vi "Diode FFT test.vi"() -> ()   [LabVIEW 2016]
uses:
  <vilib>/DAQmx/read.llb/DAQmx Read (Analog DBL 1Chan 1Samp).vi
  <vilib>/DAQmx/create/channels.llb/DAQmx Create Channel (AI-Voltage-Basic).vi
  <vilib>/DAQmx/configure/timing.llb/DAQmx Timing (Sample Clock).vi
  <vilib>/DAQmx/miscellaneous.llb/DAQmx Fill In Error Info.vi
  <vilib>/measure/maspectr.llb/FFT Power Spectrum and PSD for 1 Chan.vi
  <vilib>/measure/NI_MAPro.lvlib
panel:
  out "Waveform Graph":cluster{"f0":dbl, "df":dbl, "magnitude":dbl[]}(graph)
  out "Waveform Chart":waveform(dbl)(graph)
  in  "Stop Button":bool
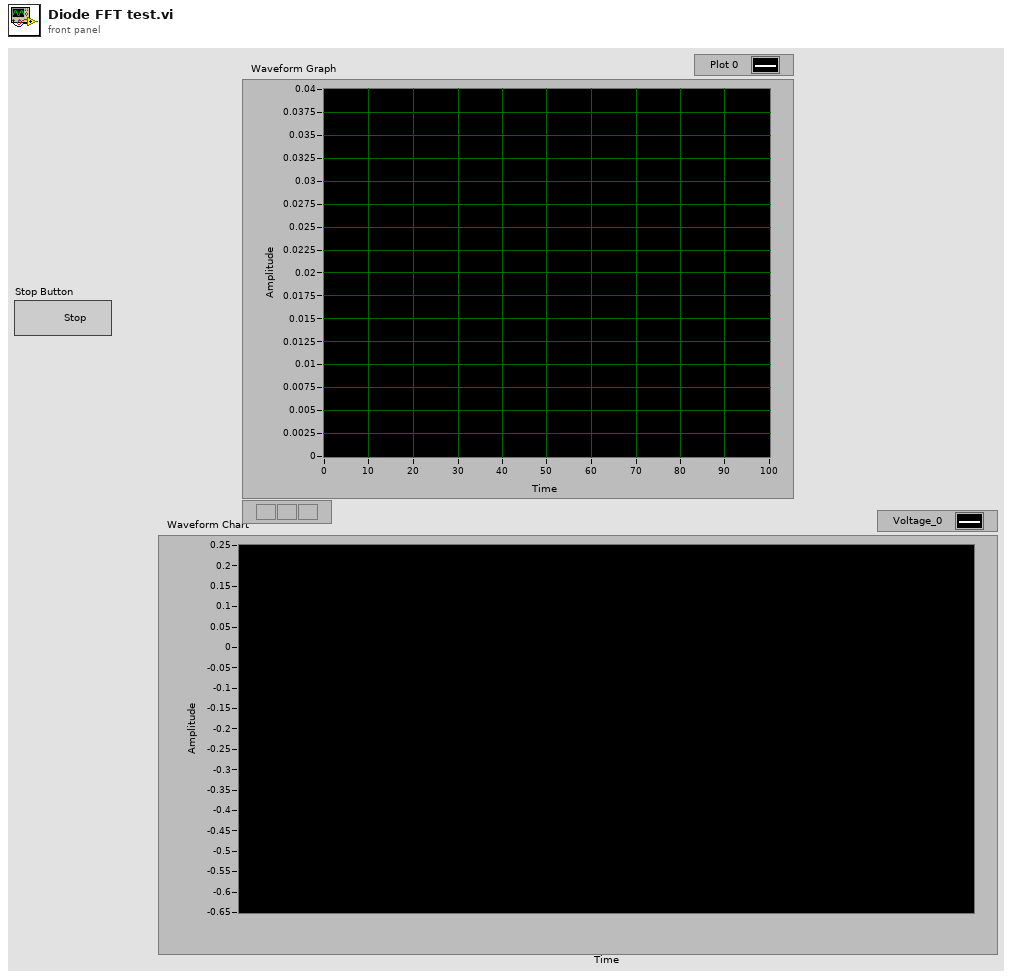
[diagram p1: front panel]
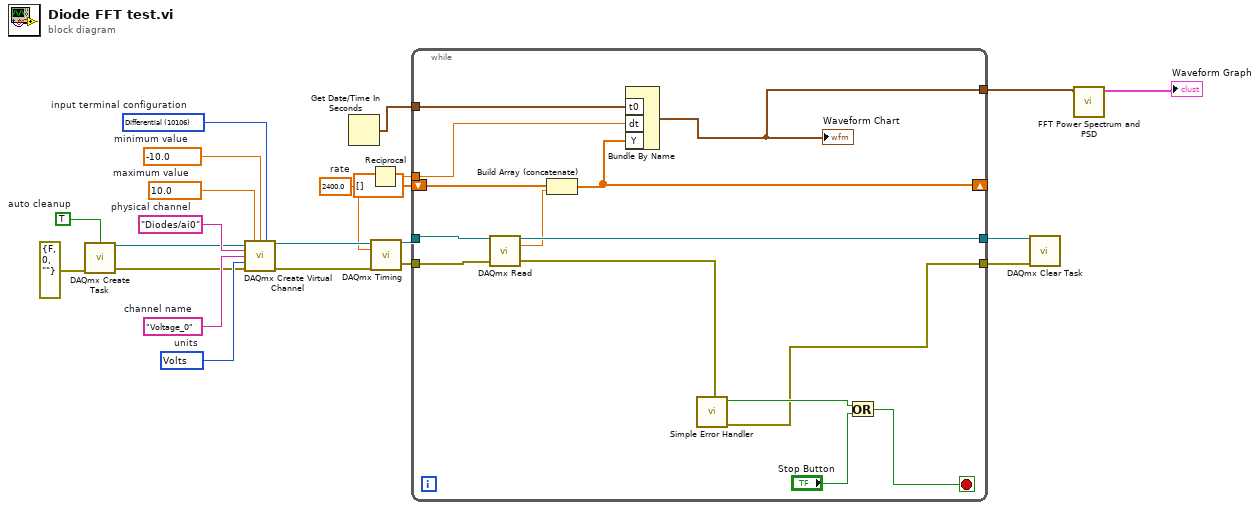
[diagram p0: block diagram]
diagram:
  w5 = 2400.0  # rate
  w13 = 10106 items=["default"=-1, "RSE"=10083, "NRSE"=10078, "Differential"=10106, "Pseudodifferential"=12529]  # input terminal configuration
  w18 = 10348 items=["Volts"=10348, "From Custom Scale"=10065]  # units
  w17 = "Voltage_0"  # channel name
  w14 = -10.0  # minimum value
  w16 = 10.0  # maximum value
  w15 = "Diodes/ai0"  # physical channel
  w20 = TRUE  # auto cleanup
  n1 = call <vilib>:"DAQmx Create Task.vi"("auto cleanup"=w20, "error in"=errorcluster {"status"=FALSE, "code"=0, "source"=""}) -> ("task out"=w11:refnum<k21>, "error out"=w12:errorcluster)  [unwired: 12 in]
  n2 = call-poly <vilib>:"DAQmx Create Virtual Channel.vi"("task in"=w11, "maximum value"=w16, "minimum value"=w14, "input terminal configuration"=w13, "physical channels"=w15, "name to assign"=w17, "units"=w18, "error in"=w12) -> ("task out"=w10:refnum<k21>, "error out"=w8:errorcluster)  [unwired: 6 in]
  n3 = Get Date/Time In Seconds() -> (seconds since 1Jan1904=w6:timestamp)
  n4 = Reciprocal(x=w5) -> (1/x=w4:dbl)
  n5 = call-poly <vilib>:"DAQmx Timing.vi"("task/channels in"=w10, "rate"=w5, "error in"=w8) -> ("task out"=w9:refnum<k21>, "error out"=w7:errorcluster)  [unwired: 11 in]
  n6 = while {
    tunnel: w7 -> [w29]
    tunnel: [w33] -> w22
    tunnel: w9 -> [w30]
    tunnel: [w32] -> w21
    tunnel: w6 -> [w28]
    tunnel: w4 -> [w27]
    shift-right: [w25] -> _
    shift-left: dbl[] [] -> [w24]
    tunnel: [w23] -> w1
    stop <- w36 stop-if-true
    n7 = call-poly <vilib>:"DAQmx Read.vi"("task/channels in"=w30, "error in"=w29) -> ("task out"=w32:refnum<k21>, "data"=w26:dbl, "error out"=w31:errorcluster)  [unwired: 11 in]
    n8 = Build Array (concatenate)(w24, w26) -> (w25:dbl[])
    n9 = Bundle By Name("t0"=w28, "dt"=w27, "Y"=w25) -> (w23:waveform(dbl))  [unwired: 1 in]
    "Waveform Chart" <- w23
    n10 = call <vilib>:"Simple Error Handler.vi"("error in (no error)"=w31) -> ("error?"=w34:bool, "error out"=w33:errorcluster)  [unwired: 4 in, 3 out]
    n11 = Or(x=w34, y="Stop Button") -> (x .or. y?=w36:bool)
  }
  n12 = call <vilib>:"DAQmx Clear Task.vi"("task in"=w21, "error in"=w22) -> ()  [unwired: 13 in, 1 out]
  n13 = call-poly <vilib>:"FFT Power Spectrum and PSD.vi"("time signal"=w1) -> ("Power Spectrum / PSD"=→"Waveform Graph":cluster{"f0":dbl, "df":dbl, "magnitude":dbl[]})  [unwired: 7 in, 3 out]
